vi "Do.vi"(8 "error in (no error)":errorcluster, 10 "Actor in":refnum<class "Actor.lvclass">, 11 "Launch New Client Proxy Msg":refnum<class "Launch New Client Proxy Msg.lvclass">) -> (0 "error out":errorcluster, 2 "Actor out":refnum<class "Actor.lvclass">)   [LabVIEW 2016, in "Server Controller.lvlib" / "Launch New Client Proxy Msg.lvclass"]
doc: "This VI delivers the message to the actor by calling the appropriate method(s) on the actor."
uses:
  Launch New Client Proxy Msg.lvclass
  <vilib>/ActorFramework/Actor/Actor.lvclass
  Server Controller.lvclass
  C:/Program Files (x86)/National Instruments/LabVIEW 2016/vi.lib/ActorFramework/Actor/Actor.lvclass
  Launch New Client Proxy Msg.lvclass/Launch New Client Proxy Msg.ctl
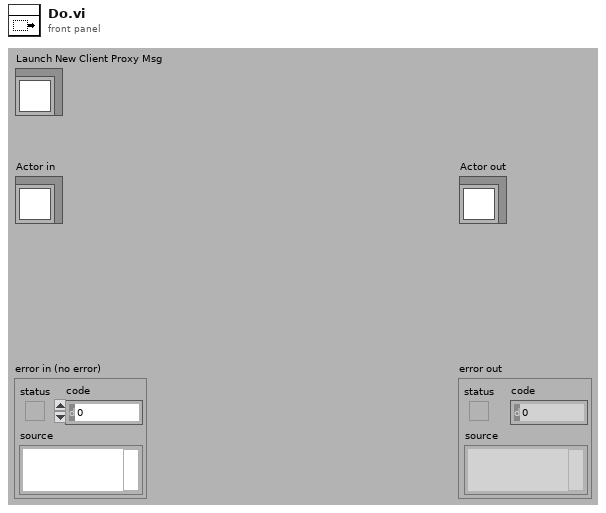
[diagram p1: front panel]
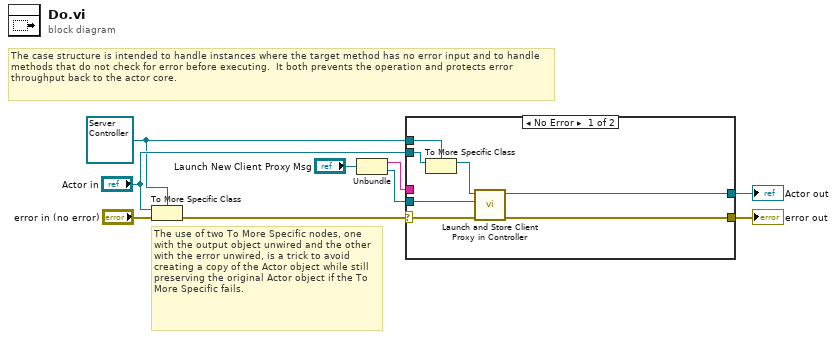
[diagram p0: block diagram]
diagram:
  w3 = refnum<class "Server Controller.lvclass"> refnum ("Actor in")
  # "The use of two To More Specific nodes, one with the output object unwired and the other with the error unwired, is a trick to avoid creating a copy of the Actor object while still preserving the original Actor object if the To More Specific fails."
  # "The case structure is intended to handle instances where the target method has no error input and to handle methods that do not check for error before executing.  It both prevents the operation and protects error throughput back to the actor core."
  n1 = To More Specific Class(target class=w3, reference="Actor in", error in="error in (no error)") -> (error out=w7:errorcluster)  [unwired: 1 out]
  n2 = Unbundle("Launch New Client Proxy Msg") -> (w2:string, w1:refnum<class "Client Proxy LNA.lvclass">)
  n3 = case shown="No Error" w7 {
    selector: w7 -> [w12 w18]
    tunnel: [w10 w18] -> w6
    tunnel: [w11 w17] -> w5
    tunnel: "Actor in" -> [w16 w17]
    tunnel: w3 -> [w15 _]
    tunnel: w2 -> [_ _]
    tunnel: w1 -> [w13 _]
    frame No Error {
      n4 = To More Specific Class(target class=w15, reference=w16) -> (specific class reference=w14:refnum<class "Server Controller.lvclass">)  [unwired: 1 in, 1 out]
      n5 = call "Launch and Store Client Proxy in Controller.vi"("error in (no error)"=w12, "Network Actor in"=w13, "Server Controller in"=w14) -> ("error out"=w10:errorcluster, "Server Controller Out"=w11:refnum<class "Server Controller.lvclass">)  [unwired: 7 in]
    }
    frame Error {
      # "If type check fails, pass the original object out again."
    }
  }
  "error out" <- w6
  "Actor out" <- w5
